vi "flecha condutor Toriginal.vi"(8 "error in (no error)":errorcluster, 11 "Dados SP":T1={"Condutor"={"Pc (N/m)"=0.0, "Mod.Young (N/m²)"=0.0, "Dil.Term.c (m/°C)"=0.0, "Área  (m²)"=0.0, "Tração EDS (N)"=0.0, "Tração Torig(N)"=0.0, "Tração Talta (N)"=0.0}, "Suporte"={"Ps (N/m)"=0.0, "Es (N/m²)"=0.0, "DTc (1/°C)"=0.0, "Área sup (m²)"=0.0, "Tração EDS sup (N)"=0.0, "Tração AT sup (N)"=0.0, "Flecha sup AT (m)"=0.0}, "Projeto"={"Temp. EDS (°C)"=0.0, "Lim.original (°C)"=0.0, "Lim.extend. (°C)"=0.0, "N. cabo/fase"=1.0}, "Vetor de dados"={"Coor.X.esp"=[], "Coor.Y.Esp."=[], "Sub.vao X"=[], "Sub.vao Y"=[], "CoordY.sup"=[], "CoordX.sup"=[]}, "Subvão"={"N. Esp."=0.0, "F.lim (m)"=0.0, "Ext.calc"=0.0, "Ext.definido"=0.0, "Comp.cabo"=0.0, "Ext.55%"=0.0, "Tração sub\nAT (N)"=0.0, "Ext.sel."=0.0, "Flecha lim.\ncalc (m)"=0.0}, "Vão"={"Extensão (m)"=0.0, "Desnivel (m)"=0.0, "Ext.Lim sub (m)"=0.0, "Flecha à 60 °C"=0.0}} {"Projeto"."N. cabo/fase" min=1.0 max=8.0 step=1.0 format="%#_1f"}) -> (0 "error out":errorcluster, 3 "Dados SP Out":T1={"Condutor"={"Pc (N/m)"=0.0, "Mod.Young (N/m²)"=0.0, "Dil.Term.c (m/°C)"=0.0, "Área  (m²)"=0.0, "Tração EDS (N)"=0.0, "Tração Torig(N)"=0.0, "Tração Talta (N)"=0.0}, "Suporte"={"Ps (N/m)"=0.0, "Es (N/m²)"=0.0, "DTc (1/°C)"=0.0, "Área sup (m²)"=0.0, "Tração EDS sup (N)"=0.0, "Tração AT sup (N)"=0.0, "Flecha sup AT (m)"=0.0}, "Projeto"={"Temp. EDS (°C)"=0.0, "Lim.original (°C)"=0.0, "Lim.extend. (°C)"=0.0, "N. cabo/fase"=1.0}, "Vetor de dados"={"Coor.X.esp"=[], "Coor.Y.Esp."=[], "Sub.vao X"=[], "Sub.vao Y"=[], "CoordY.sup"=[], "CoordX.sup"=[]}, "Subvão"={"N. Esp."=0.0, "F.lim (m)"=0.0, "Ext.calc"=0.0, "Ext.definido"=0.0, "Comp.cabo"=0.0, "Ext.55%"=0.0, "Tração sub\nAT (N)"=0.0, "Ext.sel."=0.0, "Flecha lim.\ncalc (m)"=0.0}, "Vão"={"Extensão (m)"=0.0, "Desnivel (m)"=0.0, "Ext.Lim sub (m)"=0.0, "Flecha à 60 °C"=0.0}} {"Projeto"."N. cabo/fase" min=1.0 max=8.0 step=1.0 format="%#_1f"})   [LabVIEW 2020]
uses:
  controles/SP data.ctl
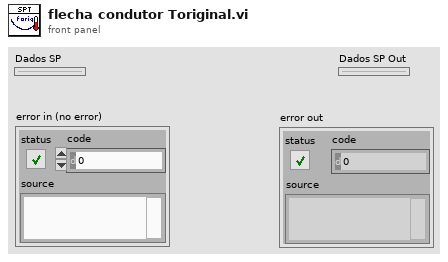
[diagram p1: front panel]
types:
  T1 = typedef "SP data.ctl" = cluster{"Condutor":cluster{"Pc (N/m)":dbl, "Mod.Young (N/m²)":dbl, "Dil.Term.c (m/°C)":dbl, "Área  (m²)":dbl, "Tração EDS (N)":dbl, "Tração Torig(N)":dbl, "Tração Talta (N)":dbl}, "Suporte":cluster{"Ps (N/m)":dbl, "Es (N/m²)":dbl, "DTc (1/°C)":dbl, "Área sup (m²)":dbl, "Tração EDS sup (N)":dbl, "Tração AT sup (N)":dbl, "Flecha sup AT (m)":dbl}, "Projeto":cluster{"Temp. EDS (°C)":dbl, "Lim.original (°C)":dbl, "Lim.extend. (°C)":dbl, "N. cabo/fase":dbl}, "Vetor de dados":cluster{"Coor.X.esp":dbl[], "Coor.Y.Esp.":dbl[], "Sub.vao X":dbl[], "Sub.vao Y":dbl[], "CoordY.sup":dbl[], "CoordX.sup":dbl[]}, "Subvão":cluster{"N. Esp.":dbl, "F.lim (m)":dbl, "Ext.calc":dbl, "Ext.definido":dbl, "Comp.cabo":dbl, "Ext.55%":dbl, "Tração sub\nAT (N)":dbl, "Ext.sel.":dbl, "Flecha lim.\ncalc (m)":dbl}, "Vão":cluster{"Extensão (m)":dbl, "Desnivel (m)":dbl, "Ext.Lim sub (m)":dbl, "Flecha à 60 °C":dbl}}
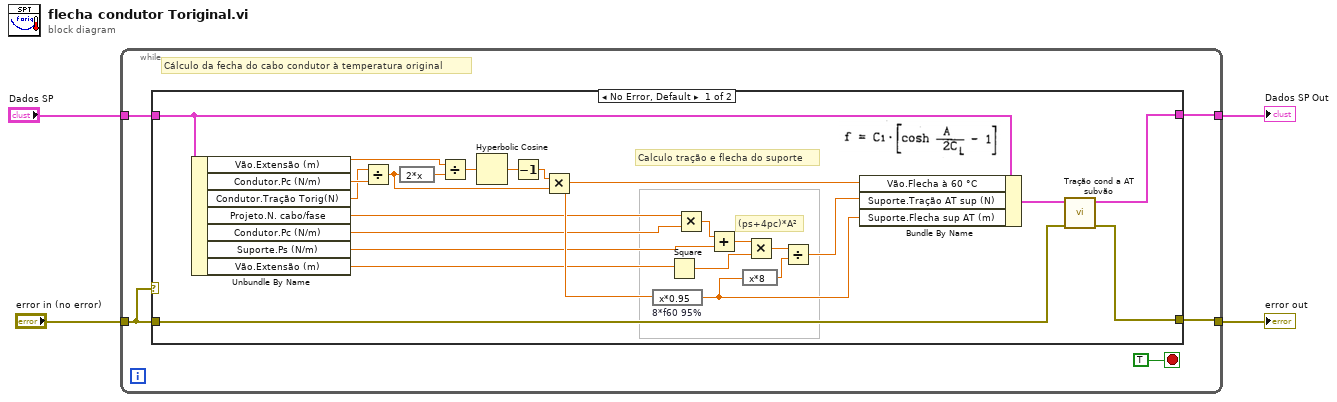
[diagram p0: block diagram]
diagram:
  n1 = while {
    tunnel: "Dados SP" -> [w9]
    tunnel: [w8] -> w3
    tunnel: "error in (no error)" -> [w6]
    tunnel: [w7] -> w1
    stop <- TRUE stop-if-true
    # "Cálculo da fecha do cabo condutor à temperatura original"
    n2 = case shown="No Error, Default" w6 {
      tunnel: w9 -> [w27 w35]
      tunnel: [w14 w35] -> w8
      tunnel: w6 -> [w13 w36]
      tunnel: [w12 w36] -> w7
      frame No Error {
        # "Calculo tração e flecha do suporte"
        # "(ps+4pc)*A²"
        n3 = Unbundle By Name(w27) -> ("Vão.Extensão (m)"=w29:dbl, "Condutor.Pc (N/m)"=w28:dbl, "Condutor.Tração Torig(N)"=w26:dbl, "Projeto.N. cabo/fase"=w23:dbl, "Condutor.Pc (N/m)"=w22:dbl, "Suporte.Ps (N/m)"=w21:dbl, "Vão.Extensão (m)"=w20:dbl)
        n4 = Divide(x=w26, y=w28) -> (x/y=w31:dbl)
        n5 = expression code="2*x"(w31) -> (w32:dbl)
        n6 = Divide(x=w29, y=w32) -> (x/y=w33:dbl)
        n7 = Hyperbolic Cosine(1:w33) -> (0:w34:dbl)
        n8 = Decrement(x=w34) -> (x-1=w30:dbl)
        n9 = Multiply(x=w30, y=w31) -> (x*y=w24:dbl)
        n10 = expression code="x*0.95" "8*f60 95%"(w24) -> (w10:dbl)
        n11 = Square(x=w20) -> (x^2=w17:dbl)
        n12 = Multiply(x=w23, y=w22) -> (x*y=w19:dbl)
        n13 = Add(x=w19, y=w21) -> (x+y=w18:dbl)
        n14 = expression code="x*8"(w10) -> (w11:dbl)
        n15 = Multiply(x=w18, y=w17) -> (x*y=w16:dbl)
        n16 = Divide(x=w16, y=w11) -> (x/y=w25:dbl)
        n17 = Bundle By Name(cluster=w27, "Vão.Flecha à 60 °C"=w24, "Suporte.Tração AT sup (N)"=w25, "Suporte.Flecha sup AT (m)"=w10) -> (w15:T1)
        n18 = call "Tração cond a AT  subvão.vi"("error in (no error)"=w13, "Dados SP"=w15) -> ("error out"=w12:errorcluster, "Dados SP Out"=w14:T1)  [unwired: 8 in]
      }
      frame Error {
      }
    }
  }
  "Dados SP Out" <- w3
  "error out" <- w1
